vi "报表.vi"(5 "姓名:":string="小明", 6 "尝试次数":string, 7 "学号:":string, 8 "Error In":errorcluster caption="错误输入", 9 "path":T1={"Excel模板.path"=path "F:/LabVIEW练习/毕设/实验成绩.xls", "Word模板.path"=path "F:/LabVIEW练习/毕设/实验报告模板.doc", "ExcelS.path"=path "F:/LabVIEW练习/毕设/实验成绩.xls", "WordS.path"=path "F:/LabVIEW练习/毕设/实验报告.doc"}, 10 "动态性能指标":T2, 11 "WFGraph引用句柄":refnum<vi>) -> (0 "Error Out":errorcluster caption="错误输出")   [LabVIEW 2018]
uses:
  <vilib>/Utility/NIReport.llb/NI_report.lvclass
  <vilib>/Utility/NIReport.llb/Report Type.ctl
  <vilib>/Utility/NIReport.llb/Append Report Text (str wrap).vi
  <vilib>/Utility/NIReport.llb/NI_ReportGenerationCore.lvlib
  <vilib>/Utility/NIReport.llb/Excel/NI_Excel.lvclass
panel:
  out "error out":errorcluster caption="错误输出"
  out "report out":refnum<class "NI_report.lvclass"> caption="报表输出"
  in  "error IO":errorcluster
  in  "report in":refnum<class "NI_report.lvclass"> caption="报表输入"
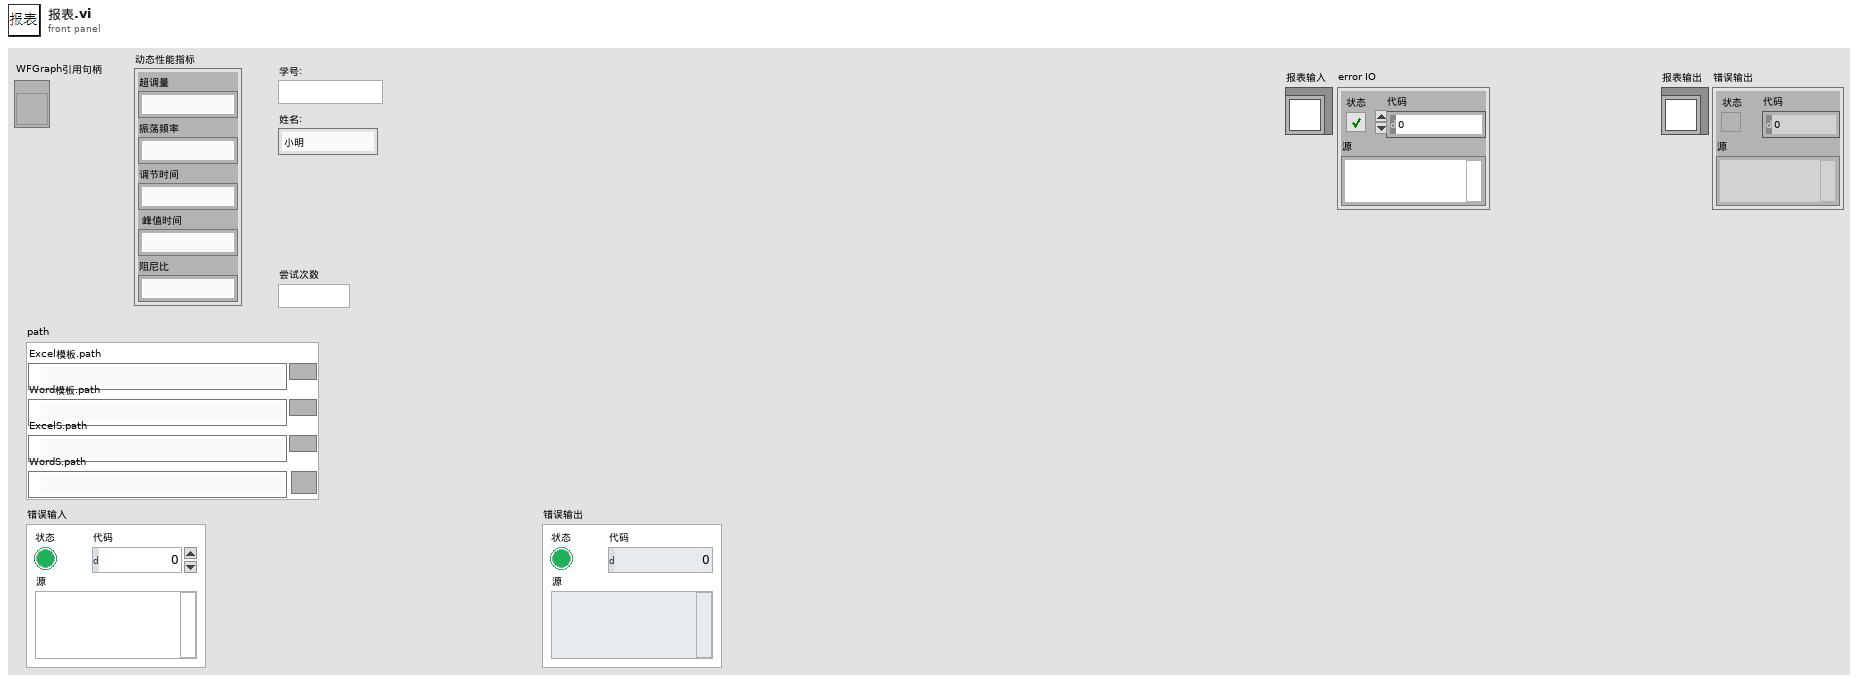
[diagram p1: front panel]
types:
  T1 = cluster{"Excel模板.path":path, "Word模板.path":path, "ExcelS.path":path, "WordS.path":path}
  T2 = cluster{"超调量":string, "振荡频率":string, "调节时间":string, " 峰值时间":string, "阻尼比 ":string}
  T3 = cluster{"pos":cluster{"row":i32, "column":i32}, "nam":string, "w":string}
  T4 = typedef "NI_ReportGenerationCore.lvlib/Report Type.ctl" = enum16{"HTML", "Word", "Excel"}
  T5 = cluster{"position (excel)":cluster{"row":i32, "column":i32}, "name (excel)":string, "bookmark (word)":string}
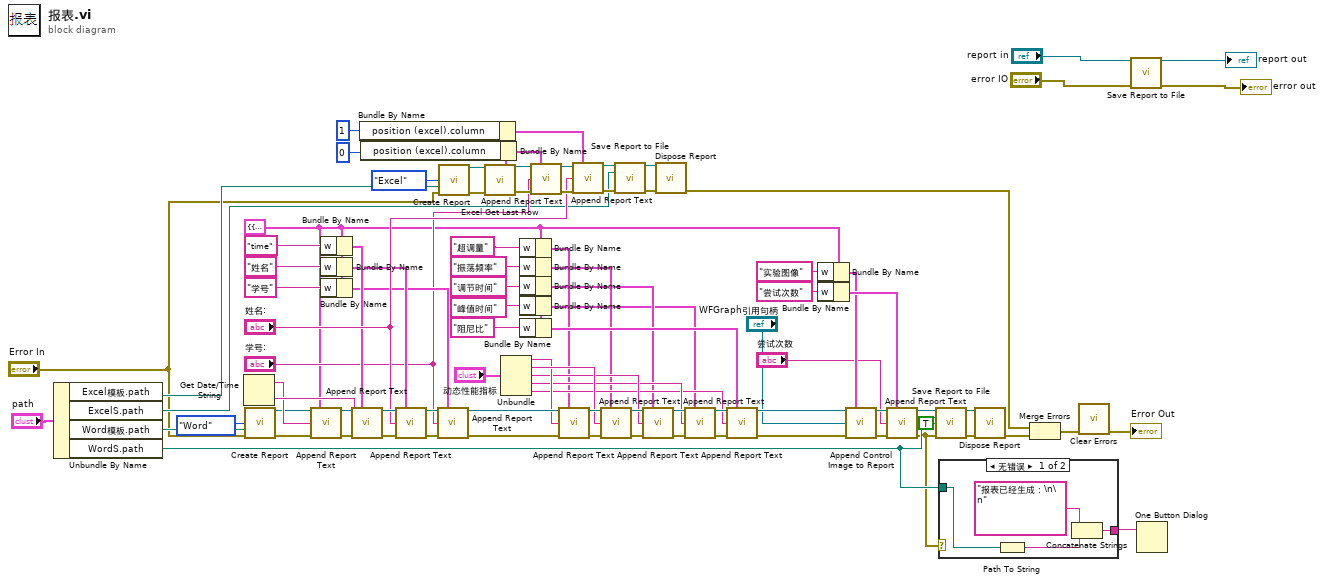
[diagram p0: block diagram]
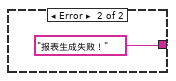
[diagram p2: hidden frame]
diagram:
  w25 = T3 {"pos"={"row"=0, "column"=0}, "nam"="", "w"="date"} ("MS Office parameters")
  n1 = Unbundle By Name("path") -> ("Excel模板.path"=w16:path, "ExcelS.path"=w15:path, "Word模板.path"=w17:path, "WordS.path"=w7:path)
  n2 = Get Date/Time String() -> (date string=w87:string, time string=w88:string)  [unwired: 3 in]
  n3 = call <vilib>:"Create Report.vi"("report type"=Report_Type."Word", "template (empty)"=w17, "error in (no error)"="Error In") -> ("report out"=w82:refnum<class "NI_report.lvclass">, "error out"=w1:errorcluster)  [unwired: 11 in]
  n4 = call-poly <vilib>:"Append Report Text.vi"("report in"=w82, "MS Office parameters"=w25, "text"=w87, "error in (no error)"=w1) -> ("report out"=w83:refnum<class "NI_report.lvclass">, "error out"=w84:errorcluster)  [unwired: 8 in, 2 out]
  n5 = Bundle By Name(cluster=w25, "w"="time" ("bookmark (word)")) -> (w37:T3)
  n6 = Bundle By Name(cluster=w25, "w"="姓名" ("bookmark (word)")) -> (w36:T3)
  n7 = Bundle By Name(cluster=w25, "w"="学号" ("bookmark (word)")) -> (w35:T3)
  n8 = call-poly <vilib>:"Append Report Text.vi"("report in"=w83, "MS Office parameters"=w37, "text"=w88, "error in (no error)"=w84) -> ("report out"=w89:refnum<class "NI_report.lvclass">, "error out"=w90:errorcluster)  [unwired: 8 in, 2 out]
  n9 = call-poly <vilib>:"Append Report Text.vi"("report in"=w89, "MS Office parameters"=w36, "text"="姓名:", "error in (no error)"=w90) -> ("report out"=w91:refnum<class "NI_report.lvclass">, "error out"=w92:errorcluster)  [unwired: 8 in, 2 out]
  n10 = call-poly <vilib>:"Append Report Text.vi"("report in"=w91, "MS Office parameters"=w35, "text"="学号:", "error in (no error)"=w92) -> ("report out"=w80:refnum<class "NI_report.lvclass">, "error out"=w3:errorcluster)  [unwired: 8 in, 2 out]
  n11 = call <vilib>:"Create Report.vi"("report type"=Report_Type."Excel", "template (empty)"=w16, "error in (no error)"="Error In") -> ("report out"=w64:refnum<class "NI_report.lvclass">, "error out"=w63:errorcluster)  [unwired: 11 in]
  n12 = call <vilib>:"Excel Get Last Row.vi"("report in"=w64, "error in (no error)"=w63) -> ("report out"=w61:refnum<class "NI_report.lvclass">, "MS Office parameters out"=w19:T5, "error out"=w62:errorcluster)  [unwired: 11 in]
  n13 = Bundle By Name(cluster=w19, "position (excel).column"=1) -> (w29:T5)
  n14 = Bundle By Name(cluster=w19, "position (excel).column"=0) -> (w27:T5)
  n15 = Unbundle("动态性能指标") -> ("超调量"=w70:string, "振荡频率"=w71:string, "调节时间"=w69:string, "峰值时间"=w68:string, "阻尼比"=w67:string)
  n16 = Bundle By Name(cluster=w25, "w"="超调量" ("bookmark (word)")) -> (w34:T3)
  n17 = Bundle By Name(cluster=w25, "w"="振荡频率" ("bookmark (word)")) -> (w33:T3)
  n18 = Bundle By Name(cluster=w25, "w"="调节时间" ("bookmark (word)")) -> (w32:T3)
  n19 = Bundle By Name(cluster=w25, "w"="峰值时间" ("bookmark (word)")) -> (w26:T3)
  n20 = Bundle By Name(cluster=w25, "w"="阻尼比" ("bookmark (word)")) -> (w41:T3)
  n21 = call-poly <vilib>:"Append Report Text.vi"("report in"=w61, "MS Office parameters"=w27, "text"="学号:", "error in (no error)"=w62) -> ("report out"=w58:refnum<class "NI_report.lvclass">, "error out"=w57:errorcluster)  [unwired: 8 in, 2 out]
  n22 = call-poly <vilib>:"Append Report Text.vi"("report in"=w80, "MS Office parameters"=w34, "text"=w70, "error in (no error)"=w3) -> ("report out"=w79:refnum<class "NI_report.lvclass">, "error out"=w78:errorcluster)  [unwired: 8 in, 2 out]
  n23 = call-poly <vilib>:"Append Report Text.vi"("report in"=w58, "MS Office parameters"=w29, "text"="姓名:", "error in (no error)"=w57) -> ("report out"=w55:refnum<class "NI_report.lvclass">, "error out"=w54:errorcluster)  [unwired: 8 in, 2 out]
  n24 = call-poly <vilib>:"Append Report Text.vi"("report in"=w79, "MS Office parameters"=w33, "text"=w71, "error in (no error)"=w78) -> ("report out"=w77:refnum<class "NI_report.lvclass">, "error out"=w76:errorcluster)  [unwired: 8 in, 2 out]
  n25 = call-dynamic "Save Report to File.vi"("report in"=w55, "report file path"=w15, "error in (no error)"=w54) -> ("report out"=w60:refnum<class "NI_report.lvclass">, "error out"=w59:errorcluster)  [unwired: 11 in]
  n26 = call-poly <vilib>:"Append Report Text.vi"("report in"=w77, "MS Office parameters"=w32, "text"=w69, "error in (no error)"=w76) -> ("report out"=w75:refnum<class "NI_report.lvclass">, "error out"=w74:errorcluster)  [unwired: 8 in, 2 out]
  n27 = call-dynamic "Dispose Report.vi"("report in"=w60, "error in (no error)"=w59) -> ("error out"=w24:errorcluster)  [unwired: 13 in]
  n28 = call-poly <vilib>:"Append Report Text.vi"("report in"=w75, "MS Office parameters"=w26, "text"=w68, "error in (no error)"=w74) -> ("report out"=w73:refnum<class "NI_report.lvclass">, "error out"=w72:errorcluster)  [unwired: 8 in, 2 out]
  n29 = call-poly <vilib>:"Append Report Text.vi"("report in"=w73, "MS Office parameters"=w41, "text"=w67, "error in (no error)"=w72) -> ("report out"=w53:refnum<class "NI_report.lvclass">, "error out"=w5:errorcluster)  [unwired: 8 in, 2 out]
  n30 = Bundle By Name(cluster=w25, "w"="实验图像" ("bookmark (Word)")) -> (w38:T3)
  n31 = Bundle By Name(cluster=w25, "w"="尝试次数" ("bookmark (word)")) -> (w40:T3)
  n32 = call-dynamic "Append Control Image to Report.vi"("report in"=w53, "ctrl reference"="WFGraph引用句柄", "error in (no error)"=w5, "MS Office parameters"=w38) -> ("report out"=w52:refnum<class "NI_report.lvclass">, "error out"=w51:errorcluster)  [unwired: 8 in, 2 out]
  n33 = call-poly <vilib>:"Append Report Text.vi"("report in"=w52, "MS Office parameters"=w40, "text"="尝试次数", "error in (no error)"=w51) -> ("report out"=w66:refnum<class "NI_report.lvclass">, "error out"=w6:errorcluster)  [unwired: 8 in, 2 out]
  n34 = call-dynamic "Save Report to File.vi"("report in"=w66, "report file path"=w7, "prompt to replace? (F)"=TRUE, "error in (no error)"=w6) -> ("report out"=w85:refnum<class "NI_report.lvclass">, "error out"=w86:errorcluster)  [unwired: 10 in]
  n35 = case shown="无错误" w6 {
    tunnel: w7 -> [w96 _]
    tunnel: [w93 "报表生成失败！"] -> w12
    frame No Error {
      n36 = Path To String(path=w96) -> (string=w94:string)
      n37 = Concatenate Strings("报表已经生成：\n\n", w94) -> (w93:string)
    }
    frame Error {
    }
  }
  n38 = call-dynamic "Dispose Report.vi"("report in"=w85, "error in (no error)"=w86) -> ("error out"=w23:errorcluster)  [unwired: 13 in]
  n39 = Merge Errors(w24, w23) -> (w22:errorcluster)
  n40 = call <vilib>:"Clear Errors.vi"("error in (no error)"=w22) -> ("error out"=→"Error Out":errorcluster)  [unwired: 5 in, 1 out]
  n41 = call-dynamic "Save Report to File.vi"("report in"="report in", "error in (no error)"="error IO") -> ("report out"=→"report out":refnum<class "NI_report.lvclass">, "error out"=→"error out":errorcluster)  [unwired: 12 in]
  n42 = One Button Dialog(message=w12) -> ()  [unwired: 1 in, 1 out]
